vi "Write Database.vi"(8 "error in (no error)":errorcluster, 10 "Database":variant, 11 "Multi Step Database in":refnum<class "Multi Step Database.lvclass">) -> (0 "error out":errorcluster, 3 "Multi Step Database out":refnum<class "Multi Step Database.lvclass">)   [LabVIEW 2016, in "NI Generic Parser.lvlib" / "Multi Step Database.lvclass"]
uses:
  Multi Step Database.lvclass
  Multi Step Database.lvclass/Multi Step Database.ctl
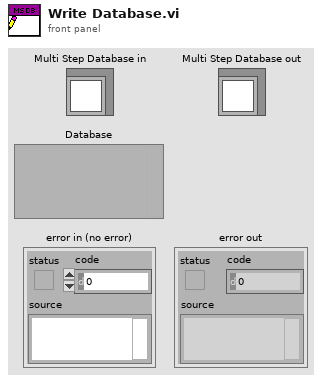
[diagram p1: front panel]
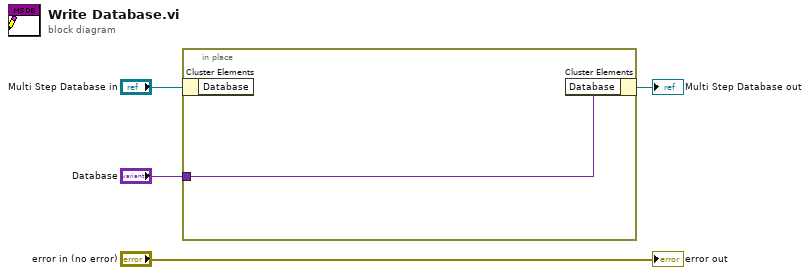
[diagram p0: block diagram]
diagram:
  n1 = in-place {
    in-place-border: "Database" -> [w5]
    n2 = in-place-cluster #1("Multi Step Database in") -> ()  [unwired: 1 out]
    n3 = in-place-cluster #1("Database"=w5) -> (→"Multi Step Database out":refnum<class "Multi Step Database.lvclass">)
  }
  "error out" <- "error in (no error)"
